vi "PathFinder.vi"(7 "All Lines":T4, 8 "Target Z":dbl format="%#_13g", 9 "Target X":dbl format="%#_13g", 11 "Posit Array":T1[](array[typedef])) -> (0 "Same Line +Dir?":bool, 1 "Path Found?":bool, 2 "Next Pos":cluster{"Line Index":i32, "Line Pos Index ":i32}, 3 "Shortest Path":T2[](array[typedef]), 4 "Index on Line":i32, 5 "Current Pos":cluster{"Line Index":i32, "Line Pos Index":i32}, 6 "Total Distance":dbl)   [LabVIEW 2014]
uses:
  Libraries/Map Data Folder/All-Lines.ctl
  Libraries/Map Data Folder/LineCluster.ctl
  Libraries/Map Data Folder/LineConnection.ctl
  Controls/PathControl.ctl
  Controls/ShortestPath.ctl
  Libraries/Contact Data/Position.ctl
  Libraries/Map Data Folder/Map Data.lvlib
  Libraries/Contact Data/Contact Data.lvlib
panel:
  out "Distance to Next":dbl
  out "All Distances":dbl[](array[numeric])
  out "Path taken out":T3[][](array[typedef])
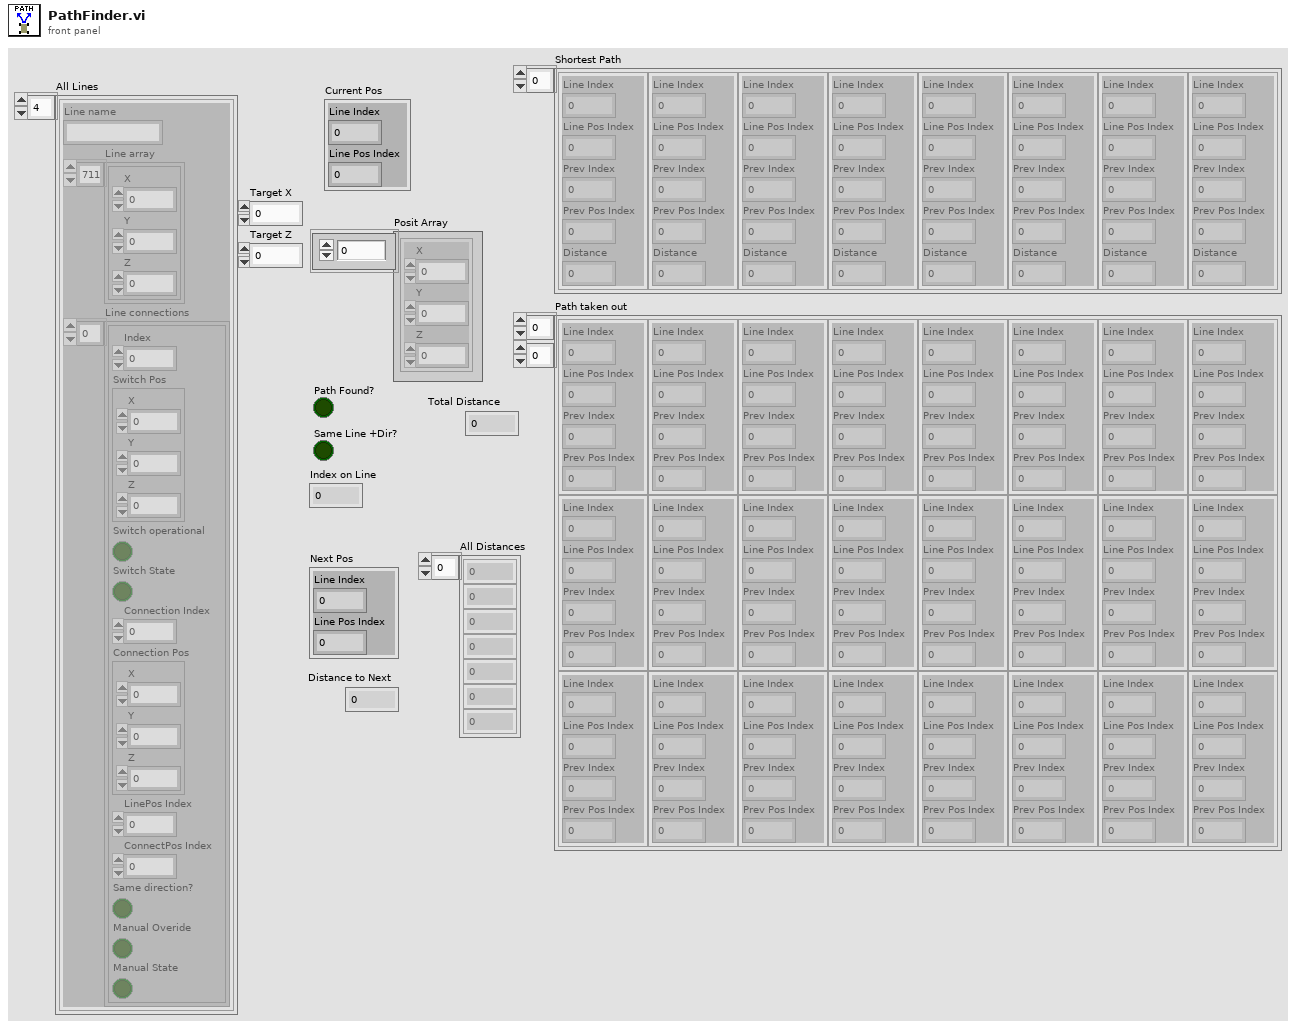
[diagram p1: front panel]
types:
  T1 = typedef "Contact Data.lvlib/Position.ctl" = cluster{"X":dbl, "Y":dbl, "Z":dbl}
  T2 = typedef "ShortestPath.ctl" = cluster{"Line Index":i32, "Line Pos Index ":i32, "Prev Index ":i32, "Prev Pos Index":i32, "Distance":dbl}
  T3 = typedef "PathControl.ctl" = cluster{"Line Index":i32, "Line Pos Index ":i32, "Prev Index ":i32, "Prev Pos Index":i32}
  T4 = typedef "Map Data.lvlib/All-Lines.ctl" = T5[]
  T5 = typedef "Map Data.lvlib/LineCluster.ctl" = cluster{"Line name":string, "Line array":cluster{"X":dbl, "Y":dbl, "Z":dbl}[], "Line connections":T6[]}
  T6 = typedef "Map Data.lvlib/LineConnection.ctl" = cluster{"Index":i32, "Switch Pos":cluster{"X":dbl, "Y":dbl, "Z":dbl}, "Switch operational":bool, "Switch State":bool, "Connection Index":i32, "Connection Pos":cluster{"X":dbl, "Y":dbl, "Z":dbl}, "LinePos Index":i32, "ConnectPos Index":i32, "Same direction?":bool, "Manual Overide":bool, "Manual State":bool}
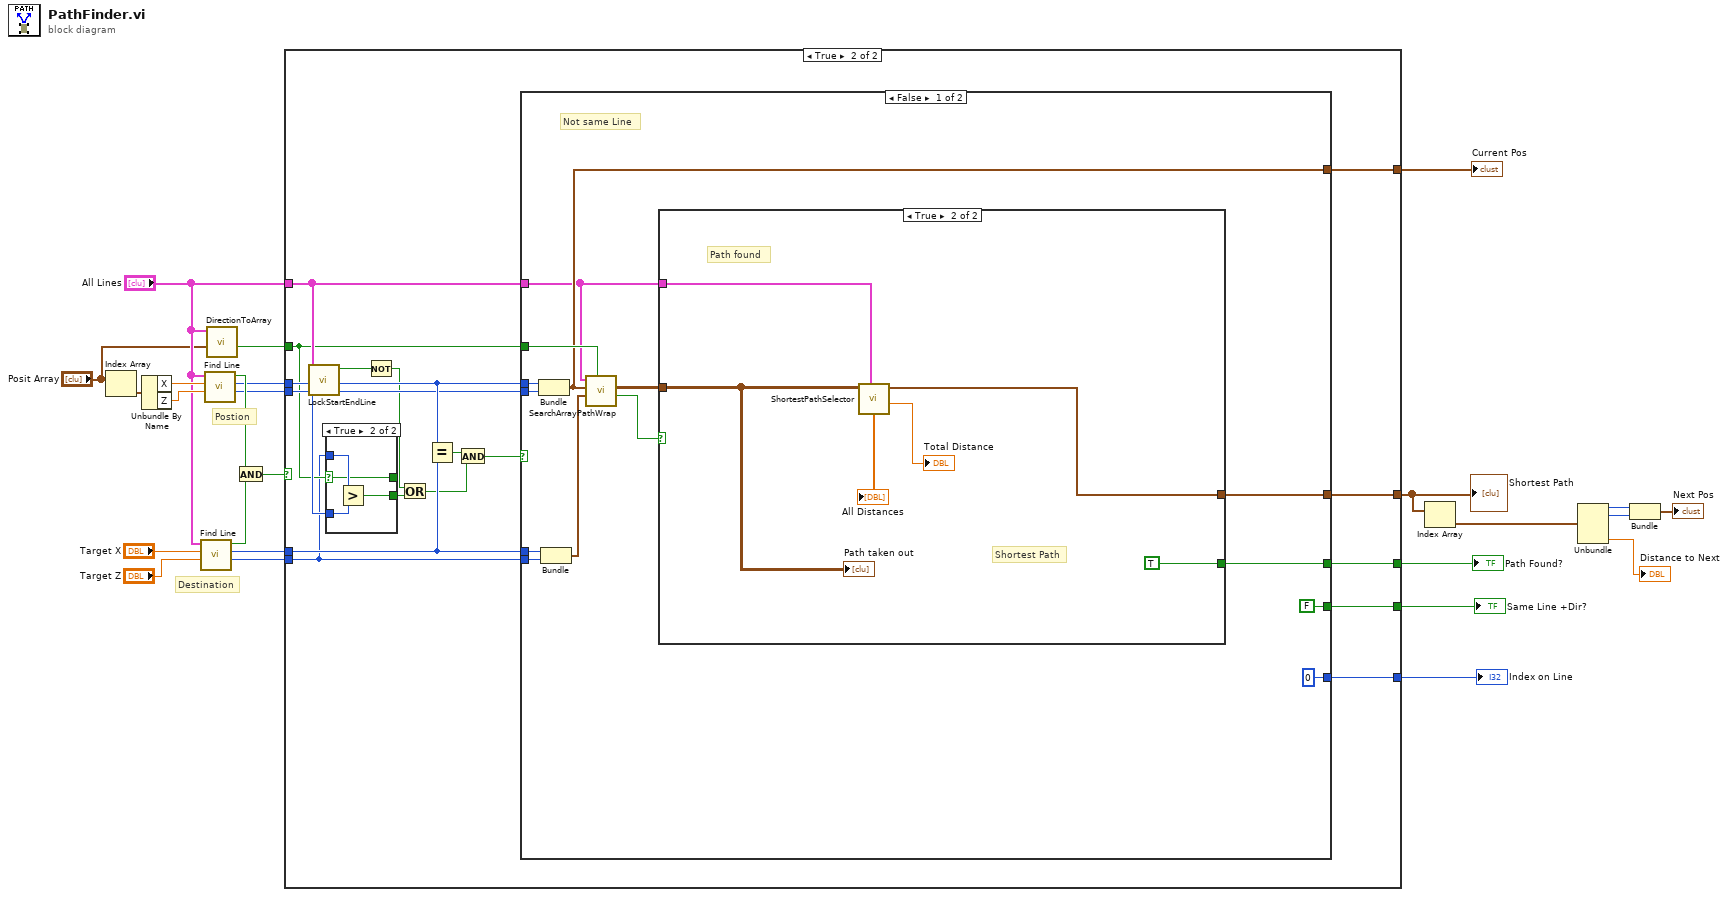
[diagram p0: block diagram]
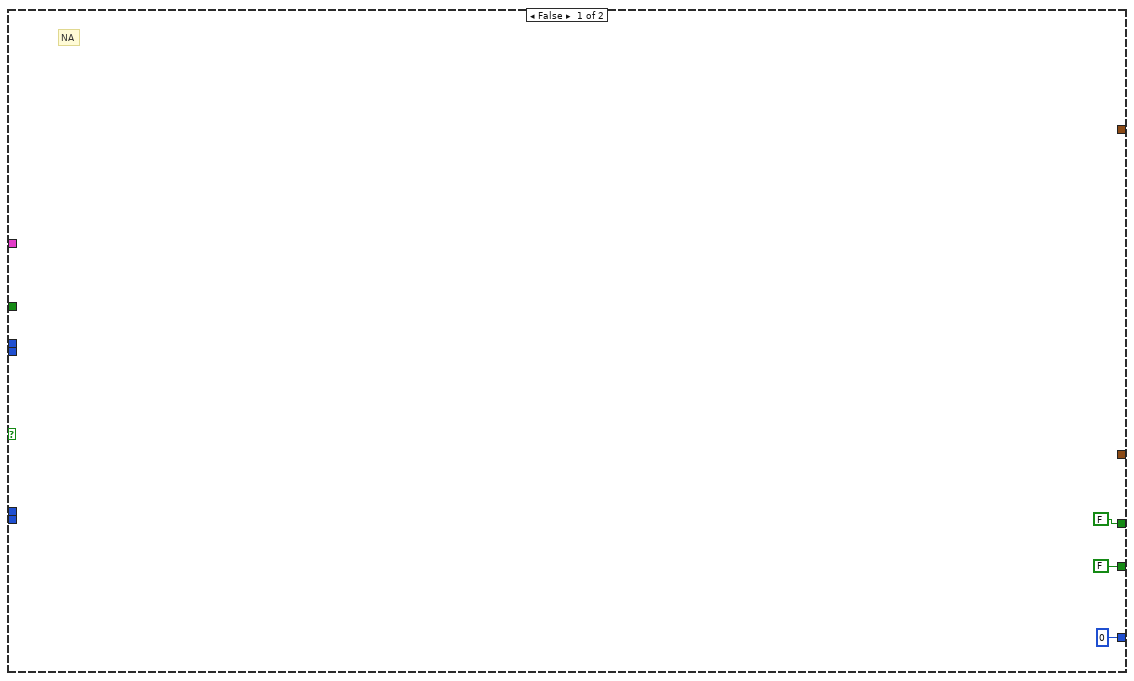
[diagram p2: hidden frame]
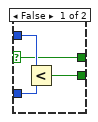
[diagram p3: hidden frame]
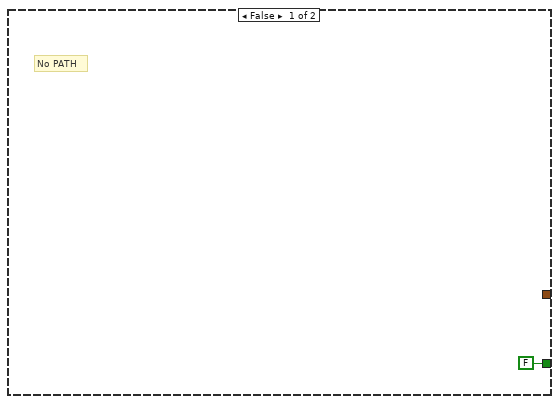
[diagram p4: hidden frame]
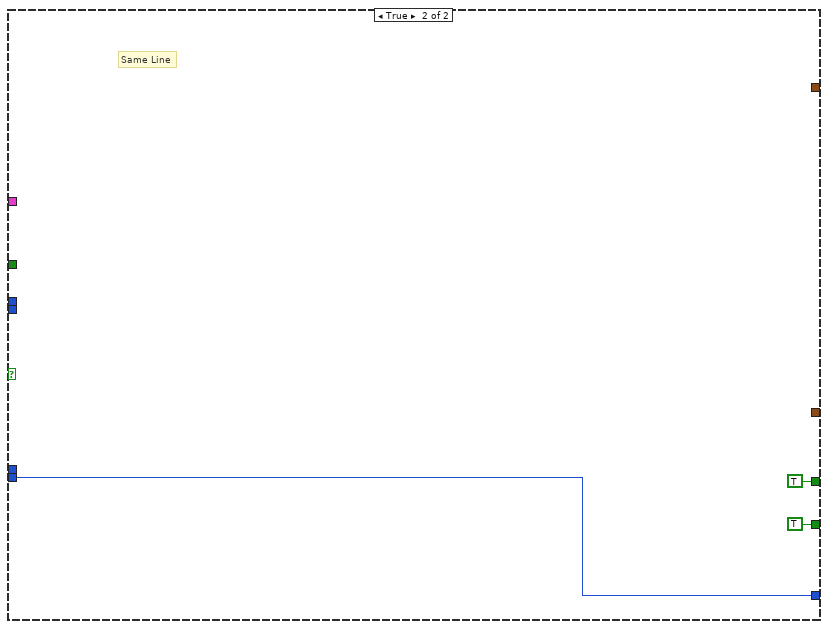
[diagram p5: hidden frame]
diagram:
  # "Postion"
  # "Destination"
  n1 = Index Array(array="Posit Array") -> (element=w13:T1)  [unwired: 1 in]
  n2 = Unbundle By Name(w13) -> ("X"=w12:dbl, "Z"=w11:dbl)
  n3 = call "Find Line.vi"("Z"="Target Z", "X"="Target X", "All Lines"="All Lines") -> ("Index on Line"=w17:i32, "Nearest Line"=w18:i32, "Line found?"=w23:bool)  [unwired: 5 in, 1 out]
  n4 = call "Find Line.vi"("Z"=w11, "X"=w12, "All Lines"="All Lines") -> ("Index on Line"=w19:i32, "Nearest Line"=w20:i32, "Line found?"=w22:bool)  [unwired: 5 in, 1 out]
  n5 = call "DirectionToArray.vi"("Posit Array"="Posit Array", "All Lines"="All Lines") -> ("Same Dir as array?"=w8:bool)  [unwired: 9 in]
  n6 = And(x=w22, y=w23) -> (x .and. y?=w21:bool)
  n7 = case shown="True" w21 {
    tunnel: "All Lines" -> [_ w40]
    tunnel: w20 -> [_ w41]
    tunnel: w19 -> [_ w39]
    tunnel: w18 -> [_ w38]
    tunnel: w17 -> [_ w30]
    tunnel: [_ w45] -> w2
    tunnel: [FALSE w44] -> w16
    tunnel: [FALSE w43] -> w15
    tunnel: [0 ("Index on Line") w42] -> w14
    tunnel: w8 -> [_ w31]
    tunnel: [_ w29] -> w3
    frame False {
      # "NA"
    }
    frame True {
      n8 = call "LockStartEndLine.vi"("index"=w41, "All Lines"=w40) -> ("Not Locked?"=w36:bool)  [unwired: 9 in]
      n9 = case shown="True" w31 {
        selector: w31 -> [w46 w50]
        tunnel: w30 -> [w49 w53]
        tunnel: w39 -> [w48 w52]
        tunnel: [w47 w51] -> w37
        tunnel: [w46 w50] -> _
        frame False {
          n10 = Less?(x=w49, y=w48) -> (x < y?=w47:bool)
        }
        frame True {
          n11 = Greater?(x=w53, y=w52) -> (0:w51:bool)
        }
      }
      n12 = Not(x=w36) -> (.not. x?=w35:bool)
      n13 = Or(x=w35, y=w37) -> (x .or. y?=w32:bool)
      n14 = Equal?(x=w41, y=w38) -> (x = y?=w33:bool)
      n15 = And(x=w33, y=w32) -> (x .and. y?=w34:bool)
      n16 = case shown="False" w34 {
        tunnel: w40 -> [w54 _]
        tunnel: w38 -> [w61 _]
        tunnel: w41 -> [w57 _]
        tunnel: [w65 _] -> w45
        tunnel: [w64 TRUE] -> w44
        tunnel: [FALSE TRUE] -> w43
        tunnel: w30 -> [w60 w75]
        tunnel: [0 ("Index on Line") w75] -> w42
        tunnel: w39 -> [w56 _]
        tunnel: w31 -> [w58 _]
        tunnel: [w55 _] -> w29
        frame False {
          # "Not same Line"
          n17 = Bundle("Nearest Line"=w57, "Index on Line"=w56) -> (w55:cluster{"Nearest Line":i32, "Index on Line":i32})  [unwired: 1 in]
          n18 = Bundle("Nearest Line"=w61, "Index on Line"=w60) -> (w59:cluster{"Nearest Line":i32, "Index on Line":i32})  [unwired: 1 in]
          n19 = call "SearchArrayPathWrap.vi"("Current Direction (T=Positive)"=w58, "Target"=w59, "Current Pos"=w55, "All Lines"=w54) -> ("Found Path?"=w67:bool, "Path taken out"=w66:T3[][])  [unwired: 6 in]
          n20 = case shown="True" w67 {
            tunnel: w66 -> [_ w73]
            tunnel: [_ w72] -> w65
            tunnel: [FALSE TRUE] -> w64
            tunnel: w54 -> [_ w69]
            frame False {
              # "No PATH"
            }
            frame True {
              # "Path found"
              # "Shortest Path"
              n21 = call "ShortestPathSelector.vi"("All Lines"=w69, "Path taken in"=w73) -> ("Total Distance"=→"Total Distance":dbl, "Shortest Path"=w72:T2[], "All Distances"=→"All Distances":dbl[])  [unwired: 7 in]
              "Path taken out" <- w73
            }
          }
        }
        frame True {
          # "Same Line"
        }
      }
    }
  }
  "Path Found?" <- w16
  "Same Line +Dir?" <- w15
  "Index on Line" <- w14
  "Shortest Path" <- w2
  "Current Pos" <- w3
  n22 = Index Array(array=w2) -> (element=w4:T2)  [unwired: 1 in]
  n23 = Unbundle(w4) -> ("Line Index"=w7:i32, "Line Pos Index"=w6:i32, "Distance"=→"Distance to Next":dbl)  [unwired: 2 out]
  n24 = Bundle("Line Index"=w7, "Line Pos Index"=w6) -> (→"Next Pos":cluster{"Line Index":i32, "Line Pos Index ":i32})  [unwired: 1 in]
